vi "DMSS.check 4 duplicate CS systems.vi"(2 "Nodes":T1[](array[typedef]) {"processes"."restartMode" items=["UNKNOWN", "MANUAL", "ONCE", "ALWAYS", "KILL", "SHUTDOWN"]}) -> (16 "duplicateSystem":bool, 17 "systemName":string)   [LabVIEW 2014, in "DMSServer.lvlib"]
doc: "Checks for duplicate CS systems"
uses:
  DMSServer.lvlib
  DMSS.node_type.ctl
  DMSS.process_type.ctl
  DomainManagementUtils/DMSU.restart_mode.ctl
  DomainManagementUtils/DMSUtils.lvlib
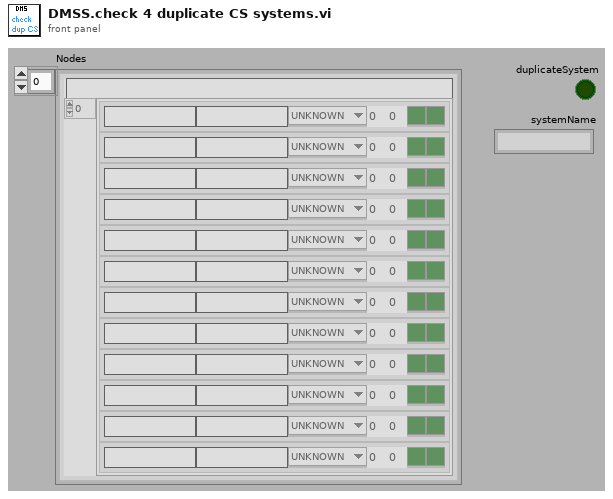
[diagram p1: front panel]
types:
  T1 = typedef "DMSServer.lvlib/DMSS.node_type.ctl" = cluster{"nodeName":string, "processes":T2[]}
  T2 = typedef "DMSServer.lvlib/DMSS.process_type.ctl" = cluster{"imageName":string, "argumentString":string, "restartMode":T3, "nOfRestart":i32, "resetRestartTimer":i32, "killOnExit":bool, "csSystem":bool}
  T3 = typedef "DMSUtils.lvlib/DMSU.restart_mode.ctl" = u16
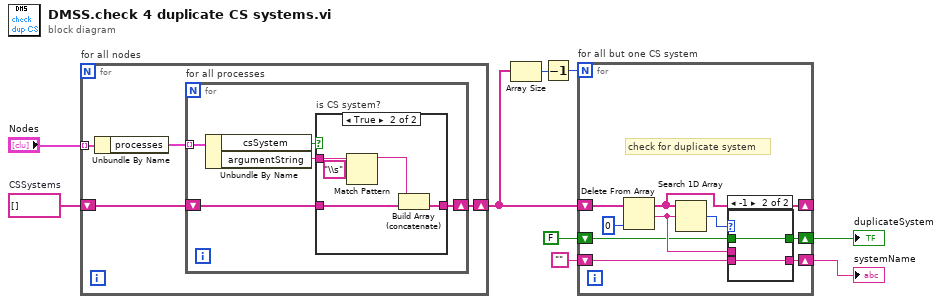
[diagram p0: block diagram]
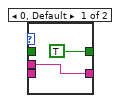
[diagram p2: hidden frame]
diagram:
  w8 = string[] []  # CSSystems
  n1 = for "for all nodes" {
    tunnel: "Nodes" -> [w13] mode=indexing
    shift-right: [w10] -> w5
    shift-left: w8 -> [w11]
    n2 = Unbundle By Name(w13) -> ("processes"=w12:T2[])
    n3 = for "for all processes" {
      tunnel: w12 -> [w18] mode=indexing
      shift-right: [w14] -> w10
      shift-left: w11 -> [w15]
      n4 = Unbundle By Name(w18) -> ("csSystem"=w17:bool, "argumentString"=w16:string)
      n5 = case "is CS system?" shown="True" w17 {
        tunnel: w16 -> [_ w23]
        tunnel: w15 -> [w19 w22]
        tunnel: [w19 w20] -> w14
        frame False {
        }
        frame True {
          n6 = Match Pattern(string=w23, regular expression="\\s") -> (before substring=w21:string)  [unwired: 1 in, 3 out]
          n7 = Build Array (concatenate)(w21, w22) -> (w20:string[])
        }
      }
    }
  }
  n8 = Array Size(array=w5) -> (size(s)=w7:i32)
  n9 = Decrement(x=w7) -> (x-1=w6:i32)
  n10 = for "for all but one CS system" {
    N: w6 -> [_]
    shift-right: [w31] -> _
    shift-left: w5 -> [w33]
    shift-right: [w29] -> w2
    shift-left: FALSE -> [w26]
    shift-right: [w27] -> w1
    shift-left: "" ("Empty String Constant") -> [w25]
    # "check for duplicate system"
    n11 = Delete From Array(array=w33, index=0) -> (deleted portion=w28:string, array with subset deleted=w31:string[])  [unwired: 1 in]
    n12 = Search 1D Array(1D array=w31, element=w28) -> (index of element=w30:i32)  [unwired: 1 in]
    n13 = case shown="-1" w30 {
      tunnel: [TRUE w37] -> w29
      tunnel: w28 -> [w34 _]
      tunnel: [w34 w36] -> w27
      tunnel: w26 -> [_ w37]
      tunnel: w25 -> [_ w36]
      frame 0, Default {
      }
      frame -1 {
      }
    }
  }
  "duplicateSystem" <- w2
  "systemName" <- w1
